vi "Read Manifold Channel Poly.vi"   [LabVIEW 2011, in "Config Manager Class.lvclass"]
uses:
  Config Manager Class.lvclass
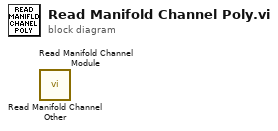
[diagram p0: block diagram]
diagram:
  n1 = call "Read Manifold Channel Other.vi"() -> ()  [unwired: 9 in, 3 out]
  n2 = call "Read Manifold Channel Module.vi"() -> ()  [unwired: 9 in, 3 out]
